vi "_easyXML_Marshal.vi"   [LabVIEW 2019]
uses:
  <vilib>/LabVIEW Open Source Project/OpenSerializer/Serializer/Serializer.lvclass
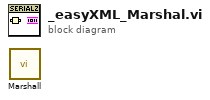
[diagram p0: block diagram]
diagram:
  n1 = call <vilib>:"Marshall.vi"() -> ()  [unwired: 9 in, 3 out]
